vi "rs3 Advanced set HDAD3.vi"(8 "error in (no error)":errorcluster, 10 "HDAD":T1, 11 "device in":u64) -> (0 "error out":errorcluster, 1 "error":u64, 3 "Dev out":u64)   [LabVIEW 2017, in "libRealSense3.lvlib"]
doc: "Sets registers inside the ASIC that affect the depth calculations.\n\nNote that for this register change to take effect the steaming must be stopped and restarted, or set before streaming."
uses:
  libRealSense3.lvlib
panel:
  # "RS3 Adv. Set HDAD 2"
  # "(C) 2017 Intel Corp.,  AGJ"
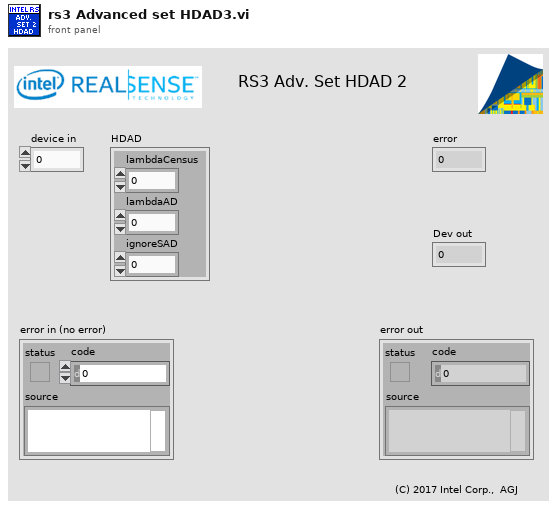
[diagram p1: front panel]
types:
  T1 = cluster{"lambdaCensus":sgl, "lambdaAD":sgl, "ignoreSAD":u32}
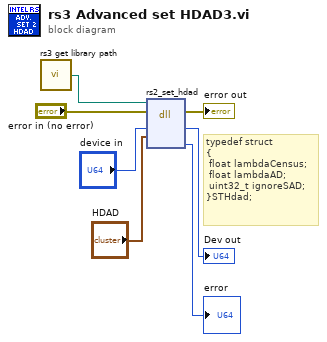
[diagram p0: block diagram]
diagram:
  # "typedef struct\n{\n\tfloat lambdaCensus;\n\tfloat lambdaAD;\n\tuint32_t ignoreSAD;\n}STHdad;"
  n1 = call "rs3 get library path.vi"() -> ("Realsense 2 Library Path"=w1:path)
  n2 = dll-call lib="C:/Users/agrunnet/Documents/libRealSense6/realsense2.dll" fn="rs2_set_hdad"(path in=w1, error in="error in (no error)", "device"="device in", "HDAD"="HDAD") -> (error out=→"error out":errorcluster, "device"=→"Dev out":u64, "error"=→"error":u64)  [unwired: 4 in, 1 out]
